vi "str.to.ob.cmd.vi"(11 "string in":string="(Time, 44700)") -> (3 "orderbook.command":T1 {"symbol" format="%.0x"; "orderId" format="%.0x"})   [LabVIEW 2020, in "fpganow.common.host.lvlib"]
uses:
  fpganow.common.host.lvlib
  fpga/orderbook.command.ctl
  fpga/orderbook.command.type.ctl
  fpga/fpganow.common.fpga.lvlib
panel:
  out "Array":string[](array[string])
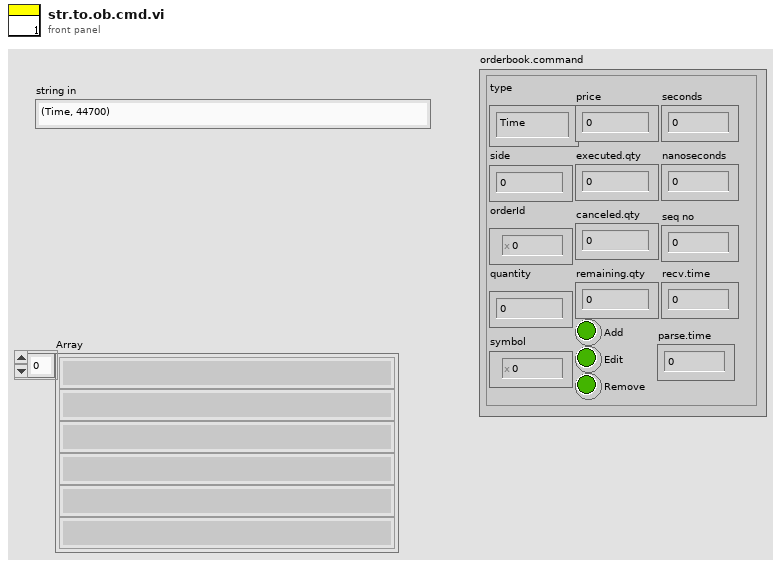
[diagram p1: front panel]
types:
  T1 = typedef "fpganow.common.fpga.lvlib/orderbook.command.ctl" = cluster{"type":T2, "side":u8, "orderId ":u64, "quantity":u32, "symbol":u64, "price":u64, "executed.qty":u32, "canceled.qty":u32, "remaining.qty":u32, "seconds":u64, "nanoseconds":u64, "Add":bool, "Edit":bool, "Remove":bool, "seq no":u32, "recv.time":u64, "parse.time":u64}
  T2 = typedef "fpganow.common.fpga.lvlib/orderbook.command.type.ctl" = enum8{"Time", "AddOrder", "OrderExecuted", "OrderExecutedAtPrice", "ReduceSize", "ModifyOrder", "DeleteOrder", "Get.Everything", "Get.All.Orders", "Get.Top"}
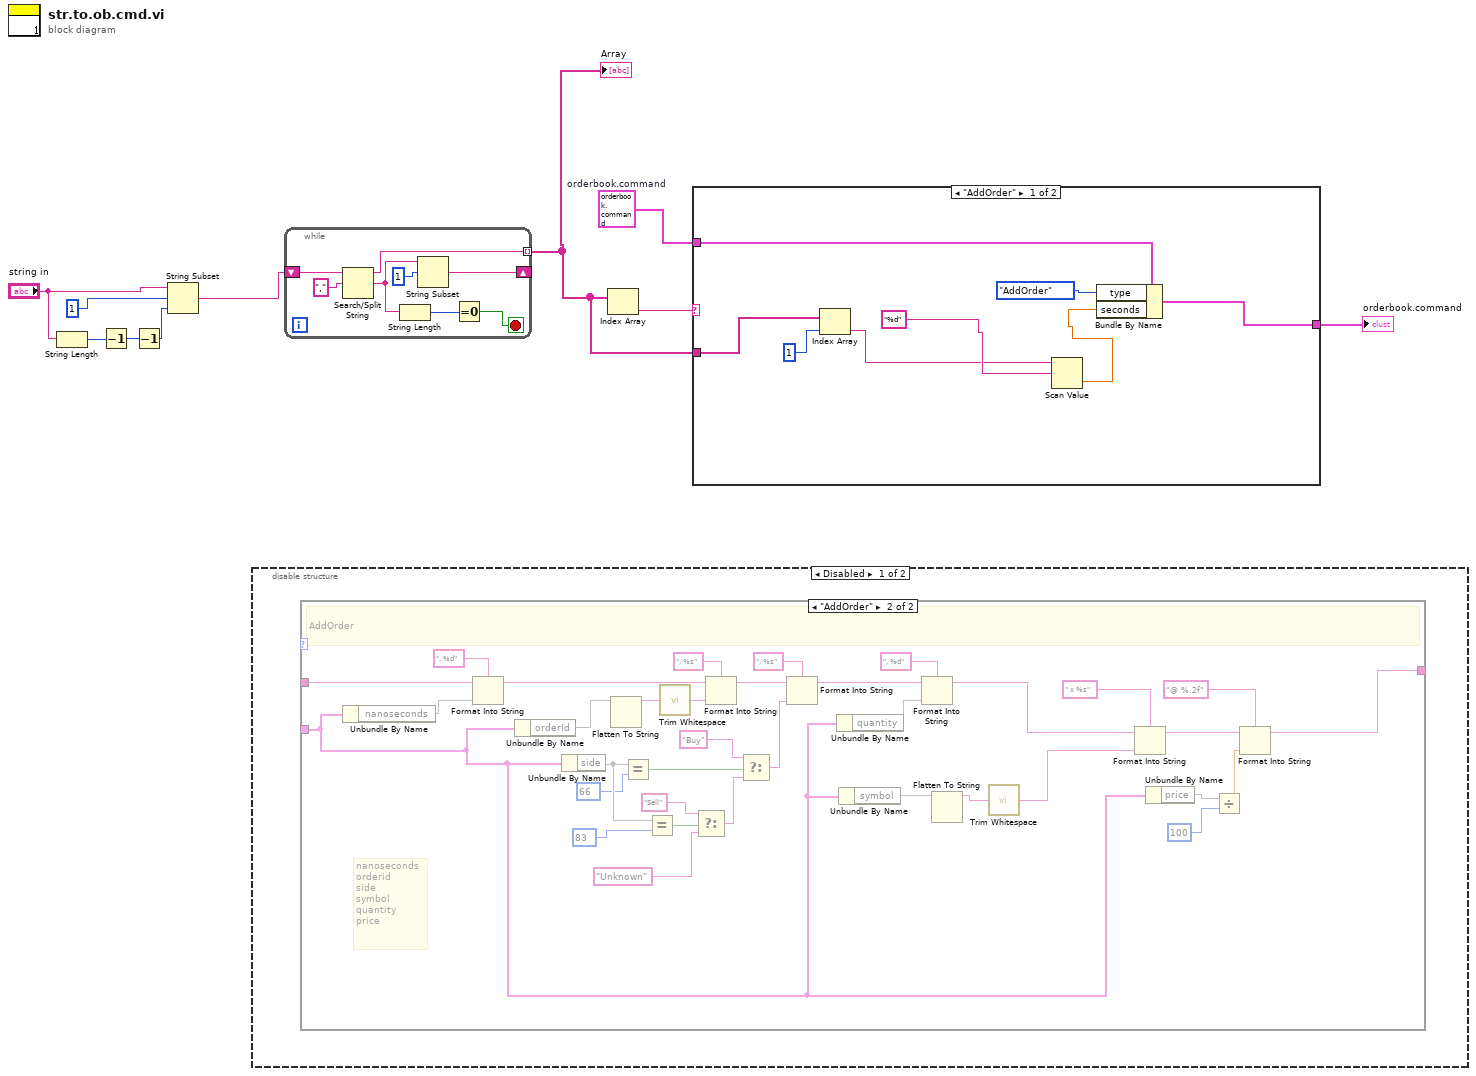
[diagram p0: block diagram]
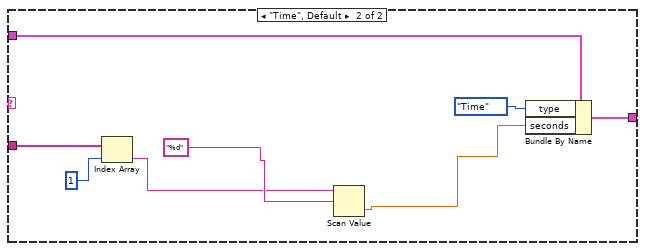
[diagram p2: hidden frame]
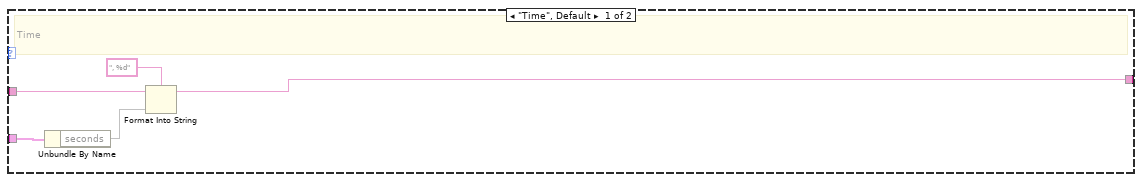
[diagram p3: hidden frame]
diagram:
  w3 = T1 {"type"=enum."Time", "side"=0, "orderId "=0, "quantity"=0, "symbol"=0, "price"=0, "executed.qty"=0, "canceled.qty"=0, "remaining.qty"=0, "seconds"=0, "nanoseconds"=0, "Add"=FALSE, "Edit"=FALSE, "Remove"=FALSE, "seq no"=0, "recv.time"=0, "parse.time"=0}  # orderbook.command
  n1 = String Length(string="string in") -> (length=w8:i32)
  n2 = Decrement(x=w8) -> (x-1=w7:i32)
  n3 = Decrement(x=w7) -> (x-1=w6:i32)
  n4 = String Subset(string="string in", offset (0)=1, length (rest)=w6) -> (substring=w5:string)
  n5 = disable-structure shown="Disabled" {
    frame Disabled {
      n6 = case shown="\"AddOrder\"" {
        selector: _ -> [_ _]
        tunnel: _ -> [w15 w22]
        tunnel: [w11 w26] -> _
        tunnel: _ -> [w12 w49]
        frame "Time", Default {
          # "Time"
          n7 = Unbundle By Name(w15) -> ("seconds"=w14)
          n8 = Format Into String(format string=", %d", initial string=w12, w14) -> (resulting string=w11:string)  [unwired: 1 in, 1 out]
        }
        frame "AddOrder" {
          # "nanoseconds\norderid\nside\nsymbol\nquantity\nprice"
          # "AddOrder"
          n9 = Unbundle By Name(w22) -> ("nanoseconds"=w50)
          n10 = Format Into String(format string=", %d", initial string=w49, w50) -> (resulting string=w46:string)  [unwired: 1 in, 1 out]
          n11 = Unbundle By Name(w22) -> ("orderId"=w16)
          n12 = Unbundle By Name(w22) -> ("side"=w43)
          n13 = Flatten To String(anything=w16) -> (data string=w18:string)  [unwired: 3 in, 2 out]
          n14 = Equal?(x=w43, y=u8 66) -> (x = y?=w37:bool)
          n15 = Equal?(x=w43, y=u8 83) -> (x = y?=w44:bool)
          n16 = call <vilib>:"Trim Whitespace.vi"("string"=w18) -> ("trimmed string"=w17:string)  [unwired: 1 in]
          n17 = Select(t="Sell", s=w44, f="Unknown") -> (s? t:f=w45:string)
          n18 = Format Into String(format string=", %s", initial string=w46, w17) -> (resulting string=w36:string)  [unwired: 1 in, 1 out]
          n19 = Select(t="Buy", s=w37, f=w45) -> (s? t:f=w35:string)
          n20 = Format Into String(format string=", %s", initial string=w36, w35) -> (resulting string=w24:string)  [unwired: 1 in, 1 out]
          n21 = Unbundle By Name(w22) -> ("quantity"=w32)
          n22 = Unbundle By Name(w22) -> ("symbol"=w21)
          n23 = Format Into String(format string=", %d", initial string=w24, w32) -> (resulting string=w23:string)  [unwired: 1 in, 1 out]
          n24 = Flatten To String(anything=w21) -> (data string=w20:string)  [unwired: 3 in, 2 out]
          n25 = call <vilib>:"Trim Whitespace.vi"("string"=w20) -> ("trimmed string"=w19:string)  [unwired: 1 in]
          n26 = Format Into String(format string=" x %s", initial string=w23, w19) -> (resulting string=w25:string)  [unwired: 1 in, 1 out]
          n27 = Unbundle By Name(w22) -> ("price"=w29)
          n28 = Divide(x=w29, y=u64 100) -> (x/y=w27:dbl)
          n29 = Format Into String(format string="@ %.2f", initial string=w25, w27) -> (resulting string=w26:string)  [unwired: 1 in, 1 out]
        }
      }
    }
    frame Enabled {
    }
  }
  n30 = while {
    shift-right: [w54] -> _
    shift-left: w5 -> [w57]
    tunnel: [w52] -> w1 mode=indexing
    stop <- w51 stop-if-true
    n31 = Search/Split String(string=w57, search string/char (-)=",") -> (substring before match=w52:string, match + rest of string=w56:string)  [unwired: 1 in, 1 out]
    n32 = String Length(string=w56) -> (length=w55:i32)
    n33 = String Subset(string=w56, offset (0)=1) -> (substring=w54:string)  [unwired: 1 in]
    n34 = Equal To 0?(x=w55) -> (x = 0?=w51:bool)
  }
  "Array" <- w1
  n35 = Index Array(array=w1) -> (element=w4:string)  [unwired: 1 in]
  n36 = case shown="\"AddOrder\"" w4 {
    tunnel: w3 -> [w65 w74]
    tunnel: [w64 w73] -> w2
    tunnel: w1 -> [w60 w71]
    frame "AddOrder" {
      n37 = Index Array(array=w60, index=1) -> (element=w61:string)
      n38 = Scan Value(string=w61, format string="%d") -> (value=w59:dbl)  [unwired: 1 in, 1 out]
      n39 = Bundle By Name(cluster=w65, "type"=orderbook.command.type."AddOrder", "seconds"=w59) -> (w64:T1)
    }
    frame "Time", Default {
      n40 = Index Array(array=w71, index=1) -> (element=w67:string)
      n41 = Scan Value(string=w67, format string="%d") -> (value=w69:dbl)  [unwired: 1 in, 1 out]
      n42 = Bundle By Name(cluster=w74, "type"=orderbook.command.type."Time", "seconds"=w69) -> (w73:T1)
    }
  }
  "orderbook.command" <- w2
